vi "Close Control References.vi"(8 "error in (no error)":errorcluster, 11 "Rename in":refnum<class "Rename.lvclass">) -> (0 "error out":errorcluster, 3 "Rename out":refnum<class "Rename.lvclass">)   [LabVIEW 2015, in "Generic Module Library.lvlib" / "Template G_Module.lvlib" / "Rename.lvclass"]
uses:
  Rename.lvclass
  Private API/Module Control Manager/Control_Mgr_Class/Controls_Mgr.lvclass
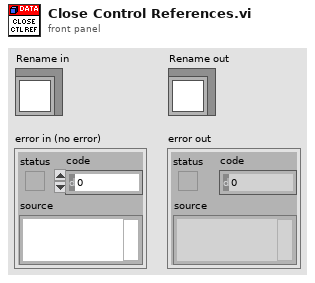
[diagram p1: front panel]
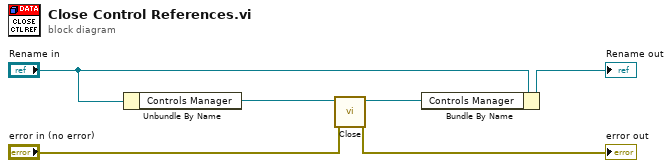
[diagram p0: block diagram]
diagram:
  n1 = Unbundle By Name("Rename in") -> ("Controls Manager"=w5:refnum<class "Controls_Mgr.lvclass">)
  n2 = call-dynamic "Close.vi"("error in (no error)"="error in (no error)", "ManageControls in"=w5) -> ("error out"=→"error out":errorcluster, "ManageControls out"=w3:refnum<class "Controls_Mgr.lvclass">)  [unwired: 8 in]
  n3 = Bundle By Name(cluster="Rename in", "Controls Manager"=w3) -> (→"Rename out":refnum<class "Rename.lvclass">)
